vi "Update Temps.vi"(0 "Lines":tag="Dev1/port0/line0:7", 5 "Inlet Temp":dbl, 7 "Outlet Temp":dbl, 9 "Product":T1=enum."LCP3", 11 "Error In":errorcluster) -> (15 "Error Out":errorcluster)   [LabVIEW 2014]
doc: "This VI generates a static analog voltage output on the line you specify."
uses:
  type defs/Product Type.ctl
  <vilib>/DAQmx/create/channels.llb/DAQmx Create Channel (AO-Voltage-Basic).vi
  <vilib>/DAQmx/write.llb/DAQmx Write (Analog 1D DBL NChan 1Samp).vi
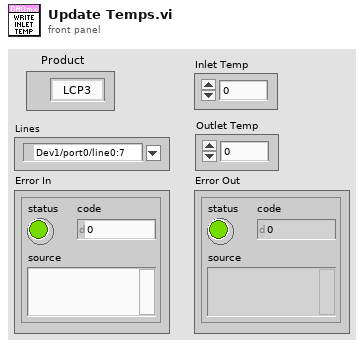
[diagram p1: front panel]
types:
  T1 = typedef "Product Type.ctl" = enum16{"Hawk", "LCP3", "2015 VA"}
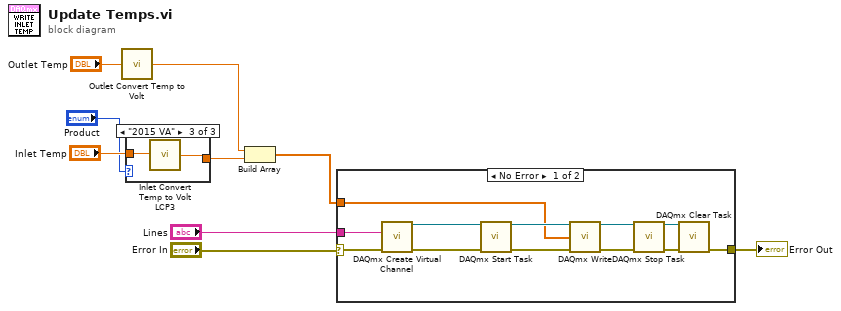
[diagram p0: block diagram]
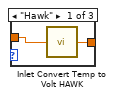
[diagram p2: hidden frame]
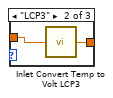
[diagram p3: hidden frame]
diagram:
  n1 = call "Outlet Convert Temp to Volt.vi"("Outlet Temperature"="Outlet Temp") -> ("Outlet Voltage"=w3:dbl)
  n2 = case shown="\"2015 VA\"" "Product" {
    tunnel: [w11 w13 w15] -> w2
    tunnel: "Inlet Temp" -> [w10 w12 w14]
    frame "Hawk" {
      n3 = call "Inlet Convert Temp to Volt HAWK.vi"("Inlet Temperature"=w10) -> ("Inlet Voltage"=w11:dbl)
    }
    frame "LCP3" {
      n4 = call "Inlet Convert Temp to Volt LCP3.vi"("Inlet Temperature"=w12) -> ("Inlet Voltage"=w13:dbl)
    }
    frame "2015 VA" {
      n5 = call "Inlet Convert Temp to Volt LCP3.vi"("Inlet Temperature"=w14) -> ("Inlet Voltage"=w15:dbl)
    }
  }
  n6 = Build Array(w3, w2) -> (w1:dbl[])
  n7 = case shown="No Error" "Error In" {
    selector: "Error In" -> [w19 w28]
    tunnel: "Lines" -> [w18 _]
    tunnel: [w17 w28] -> w7
    tunnel: w1 -> [w16 _]
    frame No Error {
      n8 = call-poly <vilib>:"DAQmx Create Virtual Channel.vi"("physical channels"=w18, "error in"=w19) -> ("task out"=w24:refnum<k21>, "error out"=w25:errorcluster)  [unwired: 12 in]
      n9 = call <vilib>:"DAQmx Start Task.vi"("task/channels in"=w24, "error in"=w25) -> ("task out"=w27:refnum<k21>, "error out"=w26:errorcluster)  [unwired: 12 in]
      n10 = call-poly <vilib>:"DAQmx Write.vi"("task/channels in"=w27, "data"=w16, "error in"=w26) -> ("task out"=w21:refnum<k21>, "error out"=w20:errorcluster)  [unwired: 10 in, 1 out]
      n11 = call <vilib>:"DAQmx Stop Task.vi"("task/channels in"=w21, "error in"=w20) -> ("task out"=w23:refnum<k21>, "error out"=w22:errorcluster)  [unwired: 12 in]
      n12 = call <vilib>:"DAQmx Clear Task.vi"("task in"=w23, "error in"=w22) -> ("error out"=w17:errorcluster)  [unwired: 13 in]
    }
    frame Error {
    }
  }
  "Error Out" <- w7
